vi "Receive Trig Command.vi"(10 "Consumer Queues in":T1) -> (0 "error out":errorcluster, 2 "Consumer Queues out":T1, 3 "Trig Process Command out":refnum<class "Generic Trig Process Command.lvclass">)   [LabVIEW 2019, in "Trig Process.lvlib" / "Generic Trig Process Command.lvclass"]
uses:
  Generic Trig Process Command.lvclass
  TS Framework/Consumer Queues.ctl
  UI Process/Generic UI Command/Generic UI Process Command.lvclass
  DAC Process/Generic DAC Command/Generic DAC Process Command.lvclass
  TS Framework/TS Framework.lvlib
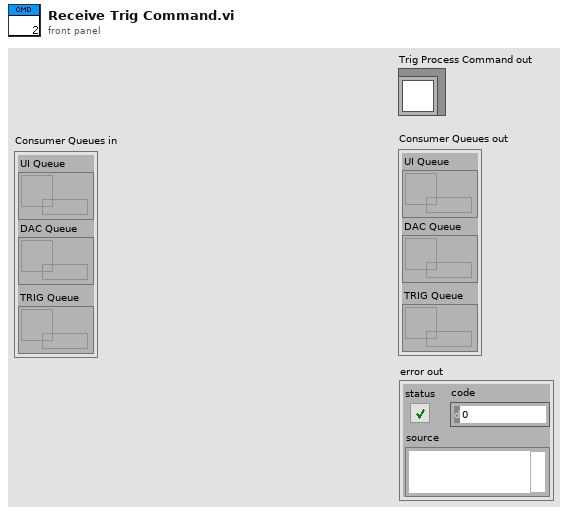
[diagram p1: front panel]
types:
  T1 = typedef "TS Framework.lvlib/Consumer Queues.ctl" = cluster{"UI Queue":refnum<queue>, "DAC Queue":refnum<queue>, "TRIG Queue":refnum<queue>}
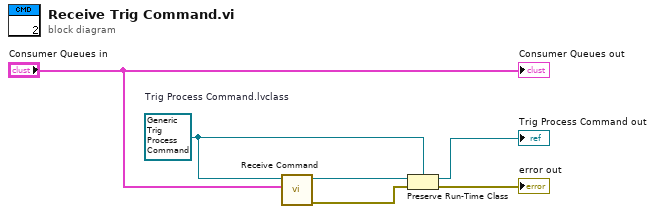
[diagram p0: block diagram]
diagram:
  w3 = refnum<class "Generic Trig Process Command.lvclass"> refnum  # Trig Process Command.lvclass
  n1 = call-dynamic "Receive Command.vi"("Consumer Queues"="Consumer Queues in", "Trig Process Command in"=w3) -> ("error out"=w4:errorcluster, "Generic Command out"=w5:refnum<class "Generic Command.lvclass">)  [unwired: 8 in]
  n2 = Preserve Run-Time Class(object in=w5, error in=w4, 2:w3) -> (object out=→"Trig Process Command out":refnum<class "Generic Trig Process Command.lvclass">, error out=→"error out":errorcluster)
  "Consumer Queues out" <- "Consumer Queues in"
